vi "Creat table.vi"(8 "query":string, 9 "table name":string, 10 "table data":string[](array[string]), 11 "Refnum in":T1) -> (2 "table data":string[](array[string]), 3 "Refnum out":T1)   [LabVIEW 2017]
uses:
  <vilib>/addons/database/Connection.llb/Conn ObjectReference.ctl
  <vilib>/addons/database/Connection.llb/Conn Execute.vi
  <vilib>/addons/database/Recordset.llb/Rec Destroy - Connection.vi
  <vilib>/addons/database/NI_Database_API.lvlib
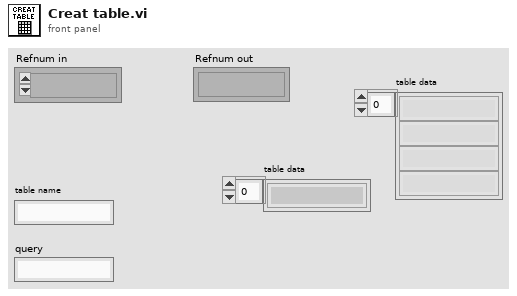
[diagram p1: front panel]
types:
  T1 = typedef "NI_Database_API.lvlib/Conn ObjectReference.ctl" = refnum<k1>
  T2 = typedef "NI_Database_API.lvlib/Rec ObjectReference.ctl" = refnum<k1>
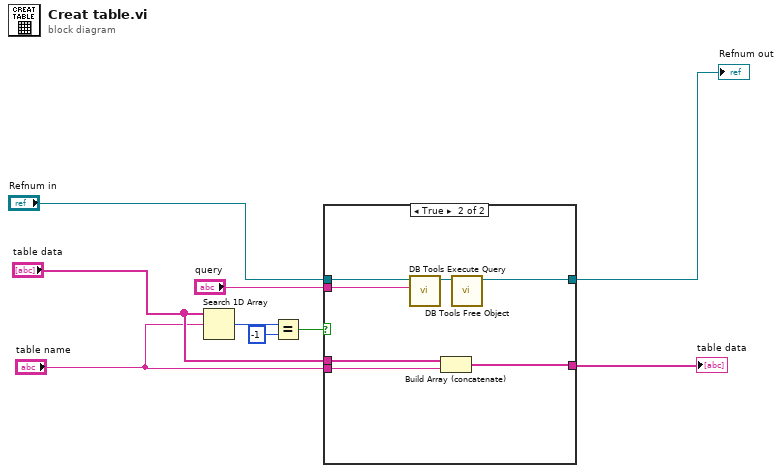
[diagram p0: block diagram]
diagram:
  n1 = Search 1D Array(1D array="table data", element="table name") -> (index of element=w4:i32)  [unwired: 1 in]
  n2 = Equal?(x=w4, y=-1) -> (x = y?=w6:bool)
  n3 = case shown="True" w6 {
    tunnel: "Refnum in" -> [w11 w18]
    tunnel: [w11 w16] -> w9
    tunnel: "query" -> [_ w15]
    tunnel: "table data" -> [w10 w14]
    tunnel: "table name" -> [_ w13]
    tunnel: [w10 w12] -> w1
    frame False {
    }
    frame True {
      n4 = call-poly <vilib>:"DB Tools Execute Query.vi"("SQL query"=w15, "connection reference"=w18) -> ("recordset reference"=w17:T2)  [unwired: 6 in, 1 out]
      n5 = Build Array (concatenate)(w14, w13) -> (w12:string[])
      n6 = call-poly <vilib>:"DB Tools Free Object.vi"("recordset reference"=w17) -> ("connection reference"=w16:T1)  [unwired: 9 in, 1 out]
    }
  }
  "Refnum out" <- w9
  "table data" <- w1
